vi "FINAL Project.vi"() -> ()   [LabVIEW 2010]
uses:
  <vilib>/express/express analysis/Spectral/XNode/ExpressSpectralMeasurementsBlockNode.xnode
  <vilib>/express/express analysis/Spectral/Block/exnSpectralBlock spectral measurements power poly.vi
  <vilib>/express/express analysis/Spectral/Block/exnSpectralBlock spectral measurements power DDT.vi
  <vilib>/ptbypt/NI_PtbyPt.lvlib
  <vilib>/Analysis/NI_AALPro.lvlib
panel:
  in  "stop":bool
  in  "Offset":dbl
  out "?":dbl(knob) scale=40.0..120.0
  out "BPM":dbl
  out "Bad":bool
  out "Good":bool
  out "Heart Rate":u32
  out "count":i32
  out "Numeric 3":dbl
  out "Amplified waveform":dynamicdata(graph)
  in  "Boolean":bool
  out "Frequency":dbl
  out "Max to Max Time":u32
  out "millisecond timer value 2":u32
  out "millisecond timer value":u32
  out "Waveform After Lowpass Filter":dynamicdata(graph)
  out "Unfiltered WaveForm":dynamicdata(graph)
  out "Amplitude":dbl
  in  "stop (F)":bool
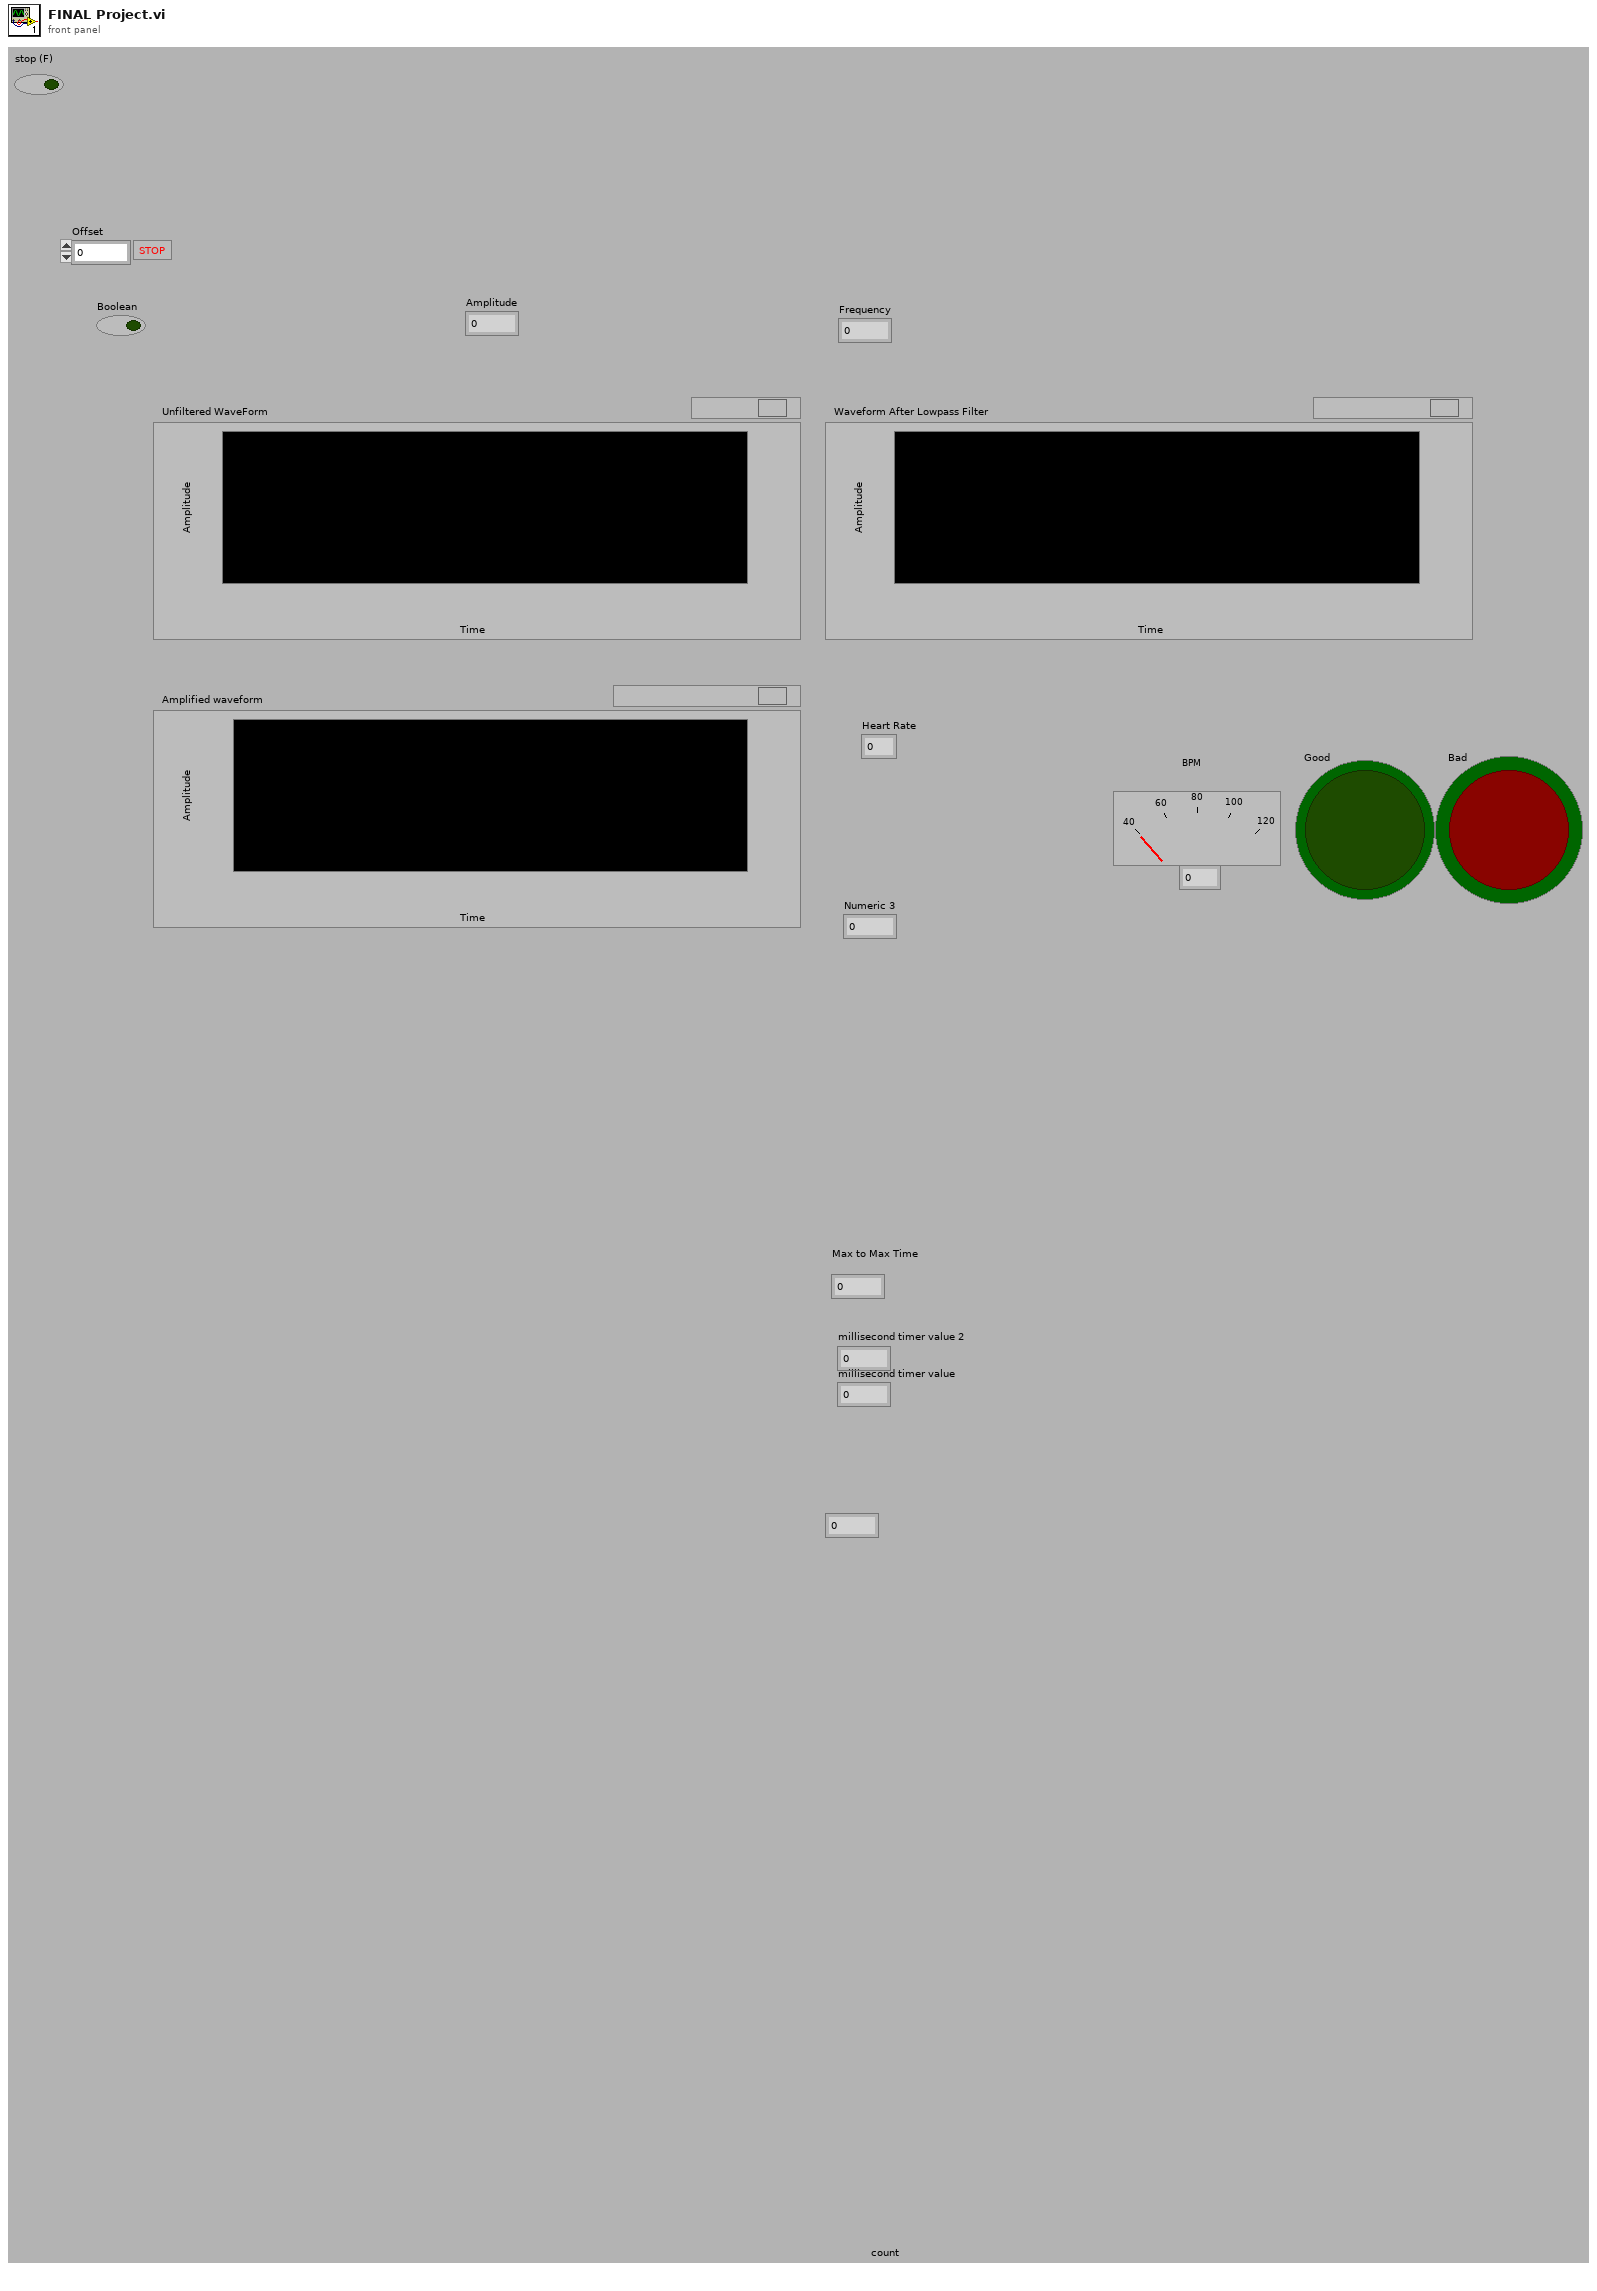
[diagram p1: front panel]
types:
  T1 = cluster{"averaging mode":u16, "weighting mode":u16, "number of averages":u32}
  T2 = cluster{"dB On (F)":bool, "unwrap phase (F)":bool, "convert to degree (F)":bool}
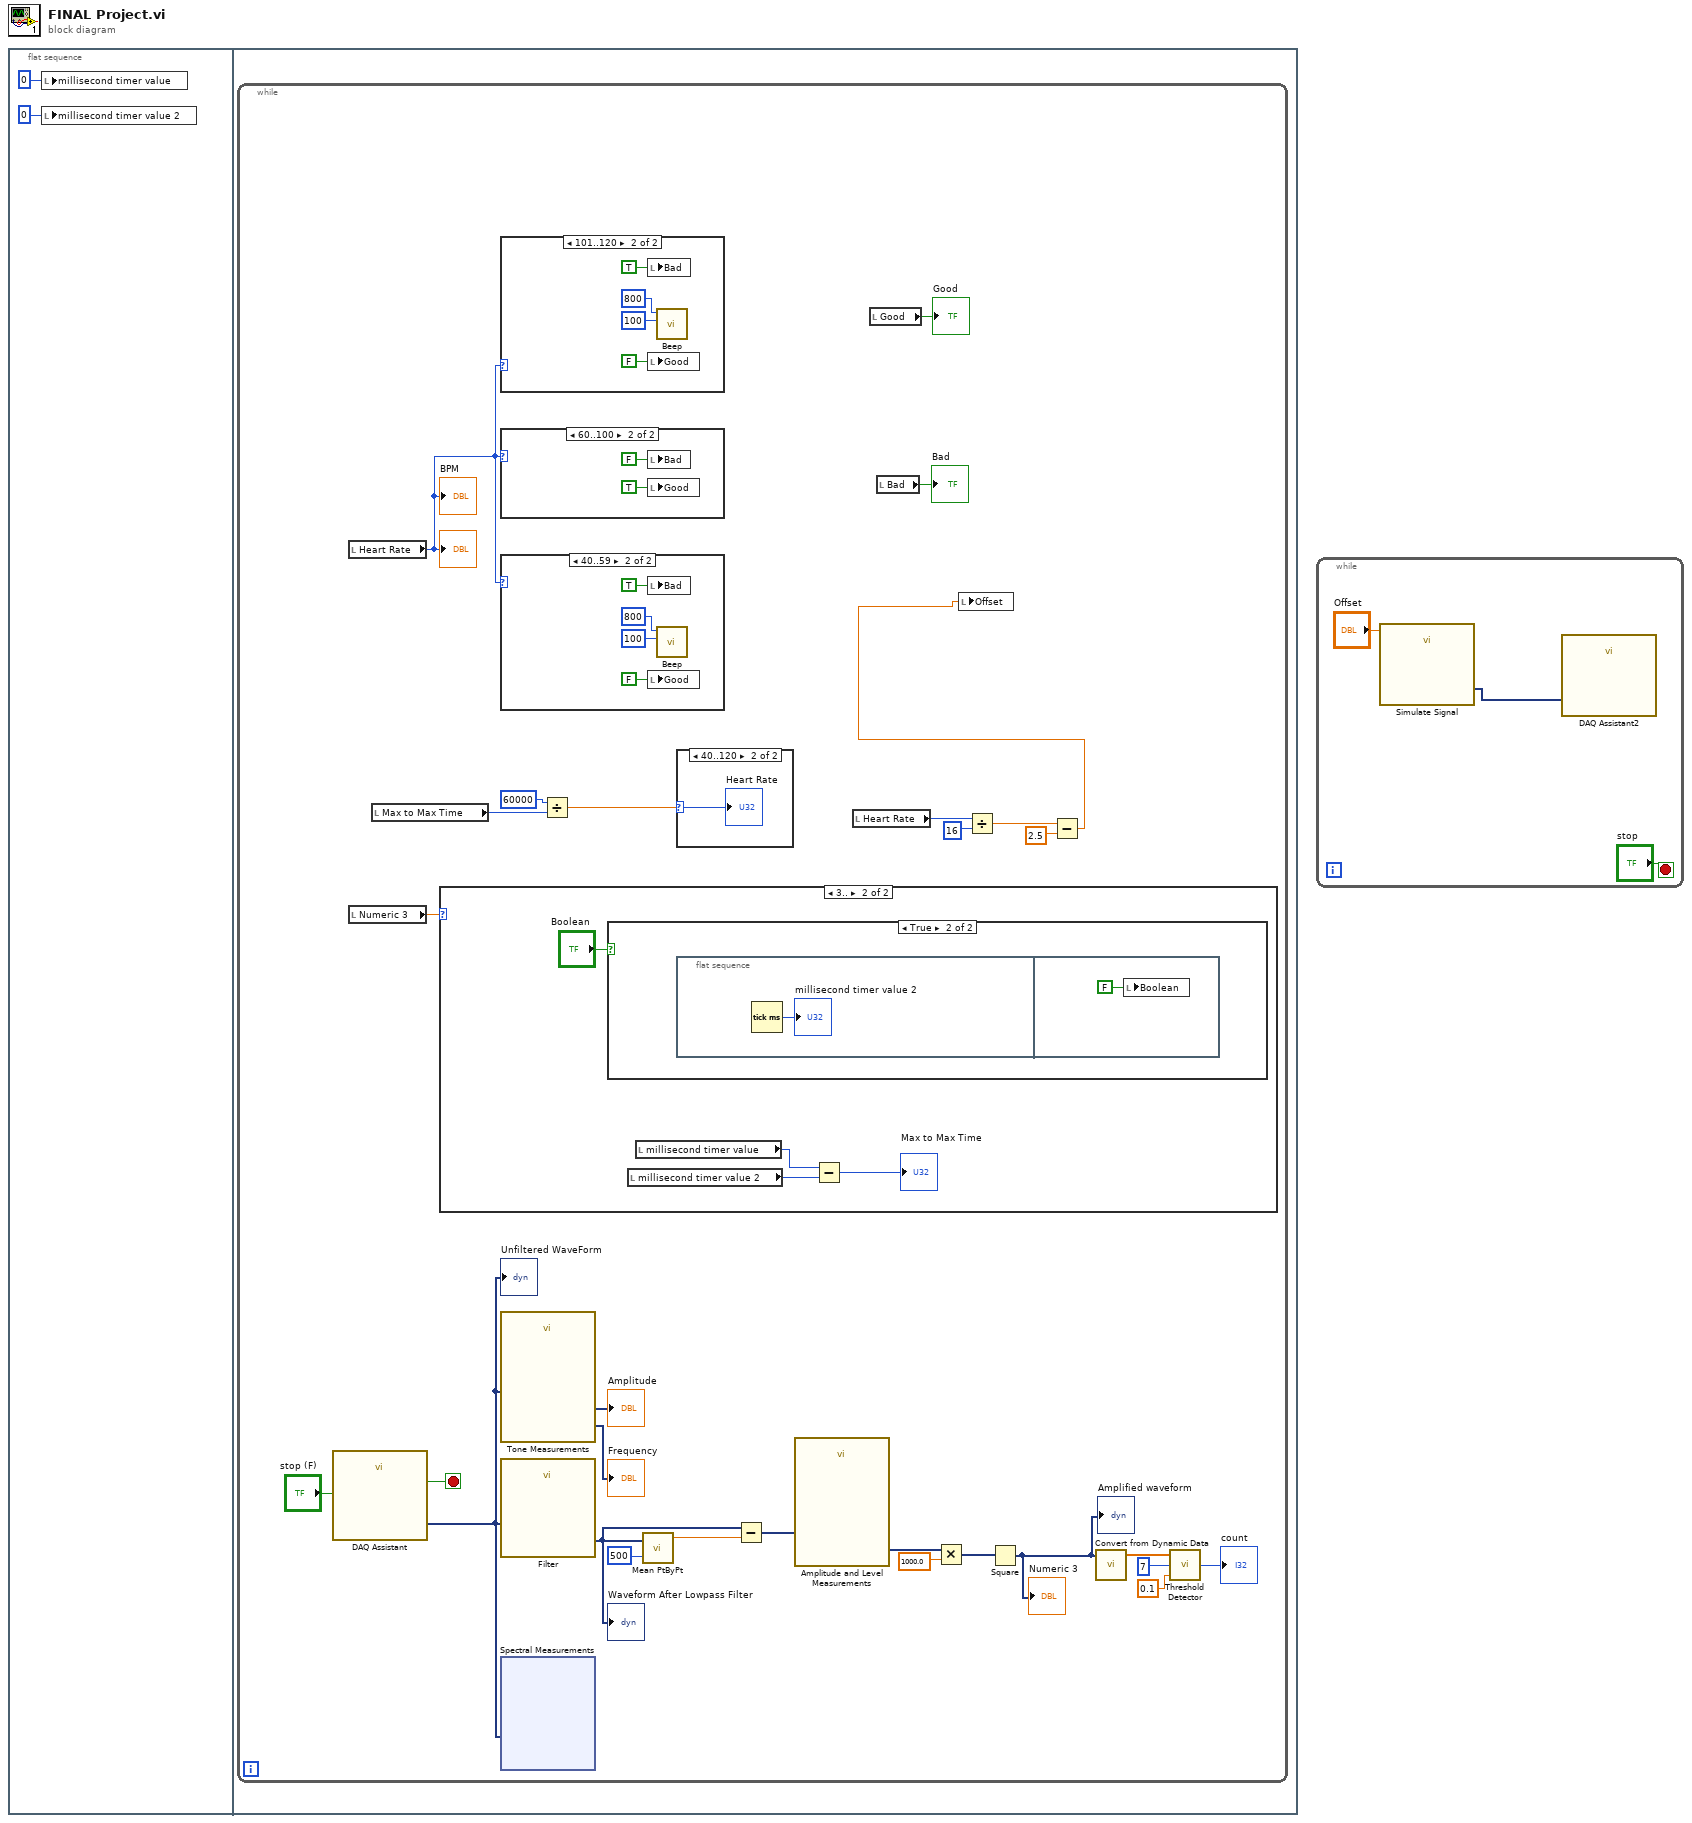
[diagram p0: block diagram]
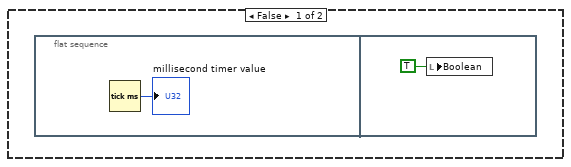
[diagram p7: hidden frame]
diagram:
  n1 = flat-sequence {
    frame #0 {
      n2 = local write "millisecond timer value"(u32 0 ("millisecond timer value")) -> ()
      n3 = local write "millisecond timer value 2"(u32 0 ("millisecond timer value 2")) -> ()
    }
    frame #1 {
      n4 = while {
        stop <- w25 stop-if-true
        n5 = call "DAQ Assistant"("stop (F)"="stop (F)") -> ("data"=w29:dynamicdata, "stopped"=w25:bool)  [unwired: 15 in, 2 out]
        "Unfiltered WaveForm" <- w29
        n6 = local read "Heart Rate"() -> (w8:u32)
        "BPM" <- w8
        "?" <- w8
        n7 = local read "Numeric 3"() -> (w14:dbl)
        n8 = local read "Max to Max Time"() -> (w11:u32)
        n9 = case shown="3.." w14 {
          frame 0, Default {
          }
          frame 3.. {
            n10 = case shown="True" "Boolean" {
              frame False {
                n11 = flat-sequence {
                  frame #0 {
                    n12 = Tick Count (ms)() -> (millisecond timer value=→"millisecond timer value":u32)
                  }
                  frame #1 {
                    n13 = local write "Boolean"(TRUE ("Boolean")) -> ()
                  }
                }
              }
              frame True {
                n14 = flat-sequence {
                  frame #0 {
                    n15 = Tick Count (ms)() -> (millisecond timer value=→"millisecond timer value 2":u32)
                  }
                  frame #1 {
                    n16 = local write "Boolean"(FALSE ("Boolean")) -> ()
                  }
                }
              }
            }
            n17 = local read "millisecond timer value 2"() -> (w44:u32)
            n18 = local read "millisecond timer value"() -> (w45:u32)
            n19 = Subtract(x=w45, y=w44) -> (x-y=→"Max to Max Time":u32)
          }
        }
        n20 = case shown="101..120" w8 {
          frame Default {
          }
          frame 101..120 {
            n21 = local write "Bad"(TRUE ("Bad")) -> ()
            n22 = local write "Good"(FALSE ("Good")) -> ()
            n23 = call <vilib>:"Beep.vi"("duration (msec)"=100, "frequency (Hz)"=800) -> ()  [unwired: 10 in]
          }
        }
        n24 = case shown="60..100" w8 {
          frame Default {
          }
          frame 60..100 {
            n25 = local write "Bad"(FALSE ("Bad")) -> ()
            n26 = local write "Good"(TRUE ("Good")) -> ()
          }
        }
        n27 = case shown="40..59" w8 {
          frame Default {
          }
          frame 40..59 {
            n28 = local write "Bad"(TRUE ("Bad")) -> ()
            n29 = local write "Good"(FALSE ("Good")) -> ()
            n30 = call <vilib>:"Beep.vi"("duration (msec)"=100, "frequency (Hz)"=800) -> ()  [unwired: 10 in]
          }
        }
        n31 = call "Tone Measurements"("Signals"=w29) -> ("Frequency"=→"Frequency":dynamicdata, "Amplitude"=→"Amplitude":dynamicdata)  [unwired: 8 in, 1 out]
        n32 = call "Filter"("Signal"=w29) -> ("Filtered Signal"=w27:dynamicdata)  [unwired: 9 in, 1 out]
        "Waveform After Lowpass Filter" <- w27
        n33 = xnode "Spectral Measurements"("Signals"=w29) -> ()  [unwired: 1 in, 2 out]
        n34 = Divide(x=60000, y=w11) -> (x/y=w13:dbl)
        n35 = call <vilib>:"Mean PtByPt.vi"("x"=w27, "sample length"=500) -> ("mean"=w26:dbl)  [unwired: 2 in, 1 out]
        n36 = case shown="40..120" w13 {
          selector: w13 -> [_ w42]
          frame Default {
          }
          frame 40..120 {
            "Heart Rate" <- w42
          }
        }
        n37 = Subtract(x=w27, y=w26) -> (x-y=w20:dynamicdata)
        n38 = call "Amplitude and Level Measurements"("Signals"=w20) -> ("Peak to Peak"=w22:dynamicdata)  [unwired: 13 in, 1 out]
        n39 = local read "Heart Rate"() -> (w7:u32)
        n40 = local read "Good"() -> (→"Good":bool)
        n41 = local read "Bad"() -> (→"Bad":bool)
        n42 = Multiply(x=w22, y=1000.0) -> (x*y=w23:dynamicdata)
        n43 = Divide(x=w7, y=16) -> (x/y=w5:dbl)
        n44 = Square(x=w23) -> (x^2=w19:dynamicdata)
        "Amplified waveform" <- w19
        "Numeric 3" <- w19
        n45 = Subtract(x=w5, y=2.5) -> (x-y=w3:dbl)
        n46 = local write "Offset"(w3) -> ()
        n47 = call "Convert from Dynamic Data"("Dynamic Data Type"=w19) -> ("Array"=w18:dbl[])  [unwired: 3 in]
        n48 = call <vilib>:"Threshold Detector.vi"("width"=0.1, "threshold"=7, "X"=w18) -> ("count"=→"count":i32)  [unwired: 2 out]
      }
    }
  }
  n49 = while {
    stop <- "stop" stop-if-true
    n50 = call "Simulate Signal"("Offset"="Offset") -> ("DC"=w61:dynamicdata)  [unwired: 13 in, 1 out]
    n51 = call "DAQ Assistant2"("data"=w61) -> ()  [unwired: 16 in, 3 out]
  }
